vi "Convert to CDO Module.vi"(8 "error in":errorcluster, 9 "SD Module in":refnum<class "SD Module.lvclass">, 10 "slot ref in":T1 format="%.0x", 11 "module in":refnum<class "Module.lvclass">) -> (0 "error out":errorcluster, 1 "SD Module out":refnum<class "SD Module.lvclass">, 2 "slot ref out":T1 format="%.0x", 3 "module out":refnum<class "Module.lvclass">)   [LabVIEW 2020, in "Scan Engine Scripting.lvlib"]
uses:
  Scan Engine Scripting.lvlib
  Modules.lvlibp/SD Module/SD Module.lvclass
  Modules/Module/Module.lvclass
  <vilib>/NI VeriStand/Custom Device API/Custom Device Item Ref.ctl
  Modules/Mode Classes/Counter Driven Output Mode/Counter Driven Output Mode.lvclass
  C:/jenkins/workspace/ercat-custom-device_release_20.4/Built/Scripting/Scan Engine/Modules/Mode Classes/Mode/Mode.lvclass
  12f3473e-bc6f-42be-bdd4-fb515759a5bc.vi
  <vilib>/NI VeriStand/Custom Device API/Custom Device API.lvlib
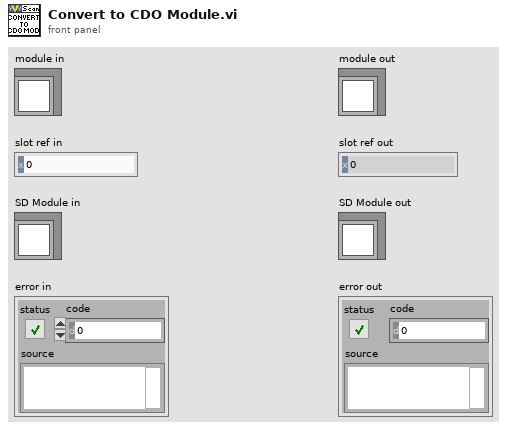
[diagram p1: front panel]
types:
  T1 = typedef "Custom Device API.lvlib/Custom Device Item Ref.ctl" = u64
  T2 = typedef "Scan Engine Scripting.lvlib/Counter Driven Output Mode.lvclass/Drive from Slot.ctl" = enum16{"Slot 1", "Slot 2", "Slot 3", "Slot 4", "Slot 5", "Slot 6", "Slot 7", "Slot 8"}
  T3 = typedef "Scan Engine Scripting.lvlib/counter driven output channel settings.ctl" = cluster{"name":string, "default value":bool, "counter driven state":T4}
  T4 = typedef "Scan Engine Scripting.lvlib/Counter Driven Output Channel.lvclass/Counter Driven State.ctl" = enum16{"Disabled", "Enabled"}
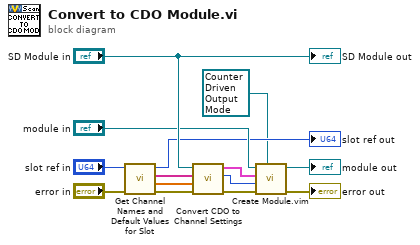
[diagram p0: block diagram]
diagram:
  n1 = call "Get Channel Names and Default Values for Slot.vi"("error in"="error in", "slot ref in"="slot ref in") -> ("error out"=w7:errorcluster, "channel default values"=w4:dbl[], "channel names"=w5:string[], "slot ref out"=→"slot ref out":T1)  [unwired: 6 in]
  n2 = call "Convert CDO to Channel Settings.vi"("error in"=w7, "channel default values"=w4, "channel names"=w5, "SD module"="SD Module in") -> ("error out"=w14:errorcluster, "drive from slot"=w1:T2, "channel settings"=w2:T3[])  [unwired: 5 in]
  n3 = call "Create Module.vim"("mode"=refnum<class "Counter Driven Output Mode.lvclass"> refnum ("Scan Engine Scripting.lvlib:Counter Driven Output Mode.lvclass"), "error in"=w14, "mode settings"=w1, "channel settings"=w2, "module in"="module in") -> ("error out"=→"error out":errorcluster, "module out"=→"module out":refnum<class "Module.lvclass">)  [unwired: 5 in]
  "SD Module out" <- "SD Module in"
